vi "FFReadCnt.vi"() -> (0 "FFCnt":u8)   [LabVIEW 2014]
uses:
  ESLSCDLL.dll
panel:
  # "how many lines are in FIFO?"
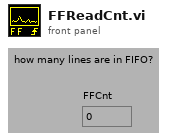
[diagram p1: front panel]
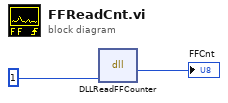
[diagram p0: block diagram]
diagram:
  n1 = dll-call lib="C:/Users/Gerhard/Documents/New64/lv/1cam/board.vis/ESLSCDLL.dll" fn="DLLReadFFCounter"("drv"=u32 1) -> ("Rückgabetyp"=→"FFCnt":u8)  [unwired: 4 in, 2 out]
